vi "Teleop Cmd Recieve.vi"(8 "error in (no error)":errorcluster, 11 "rt fifo":refnum<k33>) -> (0 "error out":errorcluster, 3 "element out":T1)   [LabVIEW 2013]
uses:
  dashboard/TeleopCmd.ctl
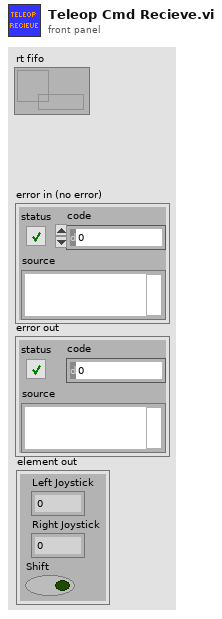
[diagram p1: front panel]
types:
  T1 = typedef "TeleopCmd.ctl" = cluster{"Left Joystick":dbl, "Right Joystick":dbl, "Shift":bool}
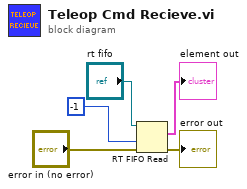
[diagram p0: block diagram]
diagram:
  n1 = RT FIFO Read(0:"rt fifo", 2:-1 ("timeout in ms (0)"), 3:"error in (no error)") -> (9:→"element out":T1, 11:→"error out":errorcluster)  [unwired: 1 in, 3 out]
